vi "getIntValue.vi"(8 "error in (no error)":errorcluster, 11 "IEnumeration in":refnum<class "IEnumeration.lvclass">) -> (0 "error out":errorcluster, 2 "Int Value out":i64, 3 "IEnumeration out":refnum<class "IEnumeration.lvclass">)   [LabVIEW 2022 SP3, in "openDAQ.lvlib" / "daqCoreTypes.lvlib" / "IEnumeration.lvclass"]
uses:
  <instrlib>/openDAQ/Public/Classes/daqCoreTypes/IEnumeration/IEnumeration.lvclass
  <instrlib>/openDAQ/Public/Classes/daqCoreTypes/IEnumeration/IEnumeration.lvclass/IEnumeration.ctl
  <instrlib>/openDAQ/Binaries/Windows/x86/copendaq32.dll
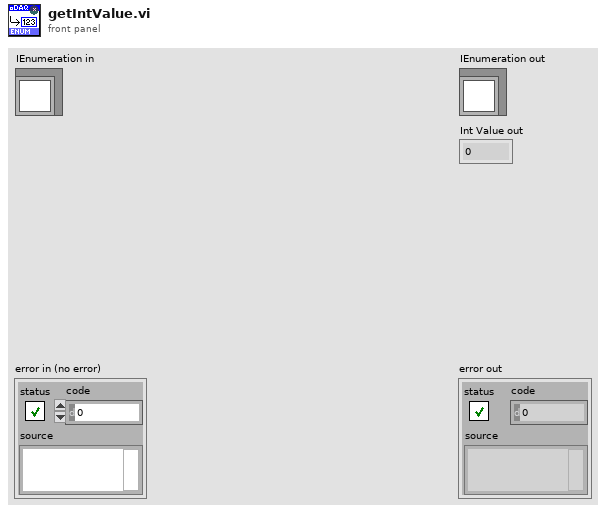
[diagram p1: front panel]
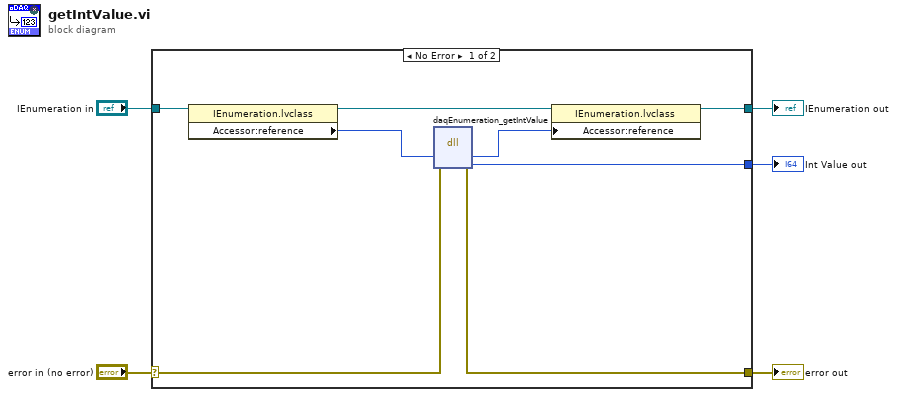
[diagram p0: block diagram]
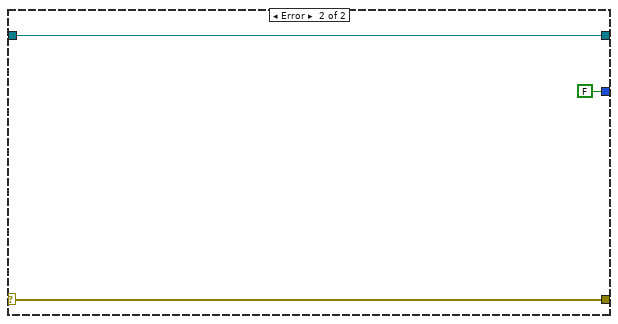
[diagram p2: hidden frame]
diagram:
  n1 = case shown="No Error" "error in (no error)" {
    selector: "error in (no error)" -> [w7 w16]
    tunnel: [w8 w16] -> w4
    tunnel: [w11 w15] -> w2
    tunnel: "IEnumeration in" -> [w13 w15]
    tunnel: [w6 FALSE] -> w1
    frame No Error {
      n2 = property class="IEnumeration.lvclass"(reference=w13) -> (reference out=w12:refnum<class "IEnumeration.lvclass">, "Accessor:reference"=w10:i64)  [unwired: 1 in, 1 out]
      n3 = dll-call lib="C:/Program Files (x86)/National Instruments/LabVIEW 2022/instr.lib/openDAQ/Binaries/Windows/x86/copendaq*.*" fn="daqEnumeration_getIntValue"(error in=w7, "enumeration"=w10) -> (error out=w8:errorcluster, "enumeration"=w9:i64, "intValue"=w6:i64)  [unwired: 4 in, 1 out]
      n4 = property class="IEnumeration.lvclass"(reference=w12, "Accessor:reference"=w9) -> (reference out=w11:refnum<class "IEnumeration.lvclass">)  [unwired: 1 in, 1 out]
    }
    frame Error {
    }
  }
  "error out" <- w4
  "IEnumeration out" <- w2
  "Int Value out" <- w1
